vi "TCP-Connect.vi"(0 "PXI Address":string, 5 "Port":i32, 9 "timeout (ms)":i32=5000, 11 "error in (no error)":errorcluster, 12 "fast response":bool) -> (4 "connection ID out":refnum<k5>, 15 "error out":errorcluster)   [LabVIEW 2020]
panel:
  out "result":i32
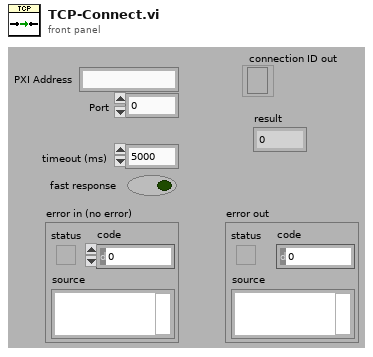
[diagram p1: front panel]
types:
  T1 = enum16{"Standard", "Buffered", "CRLF", "Immediate"}
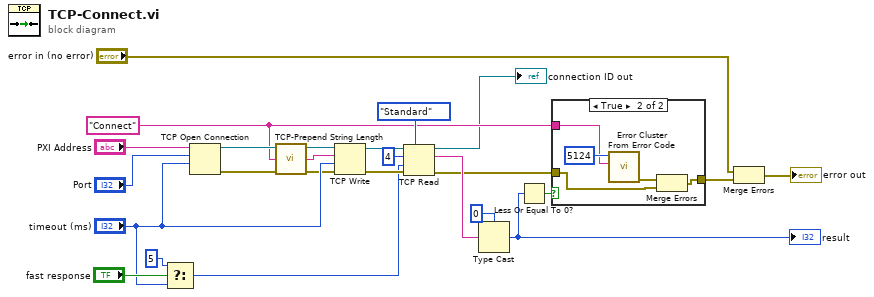
[diagram p0: block diagram]
diagram:
  w4 = "Connect" ("Command")
  n1 = Select(t=5 ("timeout ms (25000)"), s="fast response", f="timeout (ms)") -> (s? t:f=w8:i32)
  n2 = TCP Open Connection(address="PXI Address", remote port or service name="Port", timeout ms (60000)="timeout (ms)") -> (connection ID=w21:refnum<k5>, error out=w5:errorcluster)  [unwired: 2 in]
  n3 = call "TCP-Prepend String Length.vi"("Command"=w4) -> ("String"=w3:string)  [unwired: 4 in]
  n4 = TCP Write(connection ID=w21, data in=w3, error in (no error)=w5, 9:"timeout (ms)") -> (connection ID out=w20:refnum<k5>, error out=w11:errorcluster)  [unwired: 1 out]
  n5 = TCP Read(connection ID=w20, bytes to read=4, error in (no error)=w11, 7:T1."Standard" ("mode (standard)"), 9:w8) -> (connection ID out=→"connection ID out":refnum<k5>, data out=w19:string, error out=w1:errorcluster)
  n6 = Type Cast(type=0, x=w19) -> (*(type *) &x=w6:i32)
  "result" <- w6
  n7 = Less Or Equal To 0?(x=w6) -> (x <= 0?=w17:bool)
  n8 = case shown="True" w17 {
    tunnel: [w24 w26] -> w16
    tunnel: w1 -> [w24 w25]
    tunnel: w4 -> [_ w27]
    frame False {
    }
    frame True {
      n9 = call <vilib>:"Error Cluster From Error Code.vi"("error message (\"\")"=w27, "error code (0)"=5124) -> ("error out"=w29:errorcluster)  [unwired: 7 in]
      n10 = Merge Errors(w29, w25) -> (w26:errorcluster)
    }
  }
  n11 = Merge Errors("error in (no error)", w16) -> (→"error out":errorcluster)
